vi "spectral_response_main.vi"() -> ()   [LabVIEW 2018]
uses:
  typedefs/measurement_settings.ctl
  typedefs/device_details.ctl
  typedefs/state_selector.ctl
  <instrlib>/Stanford Research 830/Stanford Research 830.lvlib
panel:
  in  "Monochromator Addr in":string="ASRL7::INSTR"
  out "white bias (# of suns)":dbl
  out "integrated jsc (mA/cm^2)":dbl
  out "Application Directory":path
  out "Application Directory":string
  out "Pixel scan number":string
  out "Scan number":string
  out "Pixel data file":path
  out "Ref data filepath":path
  in  "Tab Control":enum32{"Settings", "Measurement", "Advanced"}(tab)
  in  "Load measurement settings":bool
  in  "Save device details":bool
  in  "Load device details":bool
  in  "Measurement settings":T1={"Start Wavelength (nm)"=350.0, "End Wavelength (nm)"=900.0, "Increment (nm)"=5.0, "White Bias (No. of Suns)"=1.0, "Averages per wavlength"=5.0, "Time Constant"=8, "Low Pass Filter Slope "=1, "Gain (V/A)"=50.0} {"Gain (V/A)" format="%#.2f"; "Low Pass Filter Slope" items=["6 dB/oct", "12 dB/oct", "18 db/oct", "24 dB/oct"]; "Time Constant" items=["10 us", "30 us", "100 us", "300 us", "1 ms", "3 ms", "10 ms", "30 ms", "100 ms", "300 ms", "1 s", "3 s", "10 s", "30 s", "100 s", "300 s", "1 ks", "3 ks", "10 ks", "30 ks"]; "Averages per wavlength" format="%#.2f"; "White Bias (No. of Suns)" format="%#.2f"; "End Wavelength (nm)" min=350.0 max=1100.0 format="%#.2f"; "Start Wavelength (nm)" min=350.0 max=1100.0 format="%#.2f"}
  in  "Device details":T2={"Device label"="", "Experiment Variable"="", "Variable Value"="", "Pixel"=enum."1"}
  in  "Save measurement settings":bool
  out "Username":string
  out "Experiment Name":string
  out "Zero position set":bool
  in  "Scan":bool
  in  "Initialise instruments":bool
  in  "Find Zero":bool
  in  "Calibrate ref diode":bool
  in  "Stop scan":bool
  out "TTi Power Supply":bool
  out "Pixel Selector":bool
  out "Translation Stage":bool
  out "Monochromator":bool
  in  "Exit":bool
  out "Lock-in Amplifier":bool
  out "Reference measured":bool
  in  "Stop reference":bool
  in  "Wavelength (nm)":dbl
  in  "LED current (A)":dbl=0.1 min=0.0 max=0.5
  in  "Pixel":u16=1
  out "Light on":bool
  in  "Toggle white light":bool
  in  "Lock-in address":refnum<visa-resource-name>="GPIB0::8::INSTR"
  in  "TTi QL564P":refnum<visa-resource-name>="COM6"
  in  "Set wavelenth":bool
  in  "Set switch":bool
  in  "Input Connection (0: Single-Ended Voltage)":u16(ring) items=["Single-Ended Voltage", "Differential Voltage", "1 MOhm Current Gain", "100 MOhm Current Gain"]
  in  "Tab Control 2":enum32{"Page 1"}(tab)
  out "Graph":cluster{dbl[], "eqe measurements":dbl[]}[](graph)
  out "Graph 2":cluster{dbl[], dbl[]}(graph)
  # "Spectral Response Measurement"
  # "1."
  # "2."
  # "3."
  # "4."
  # "5."
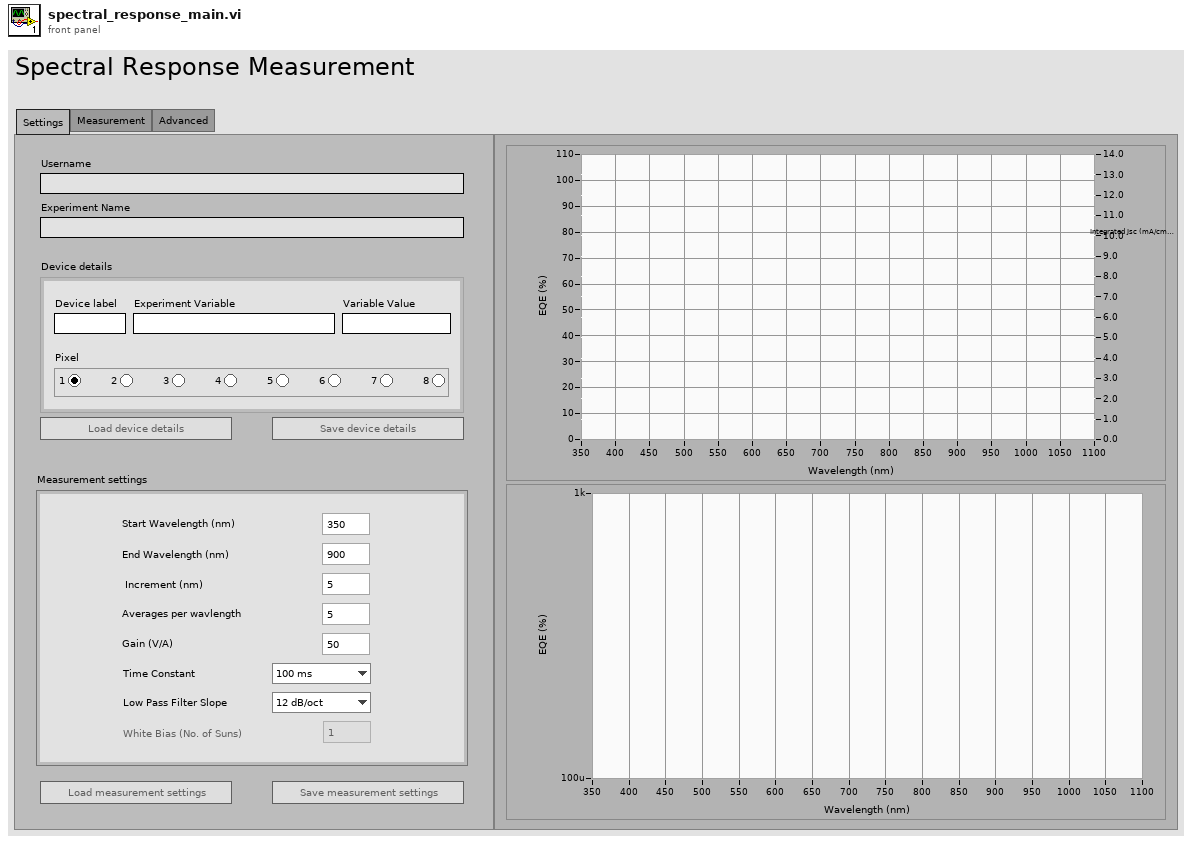
[diagram p1: front panel]
types:
  T1 = typedef "measurement_settings.ctl" = cluster{"Start Wavelength (nm)":dbl, "End Wavelength (nm)":dbl, "Increment (nm)":dbl, "White Bias (No. of Suns)":dbl, "Averages per wavlength":dbl, "Time Constant":u16, "Low Pass Filter Slope ":u16, "Gain (V/A)":dbl}
  T2 = typedef "device_details.ctl" = cluster{"Device label":string, "Experiment Variable":string, "Variable Value":string, "Pixel":enum32{"No Selection", "1", "2", "3", "4", "5", "6", "7", "8"}}
  T3 = typedef "state_selector.ctl" = enum16{"Initialise software", "Idle", "Load device details", "Save device details", "Initialise instruments", "Find zero position", "Calibrate ref diode", "Scan", "Exit"}
  T4 = enum8{"Enabled", "Disabled", "Disabled and Grayed Out"}
  T5 = cluster{"Device label":string, "Experiment Variable":string, "Variable Value":string, "Pixel":enum32{"No Selection", "1", "2", "3", "4", "5", "6", "7", "8"}}
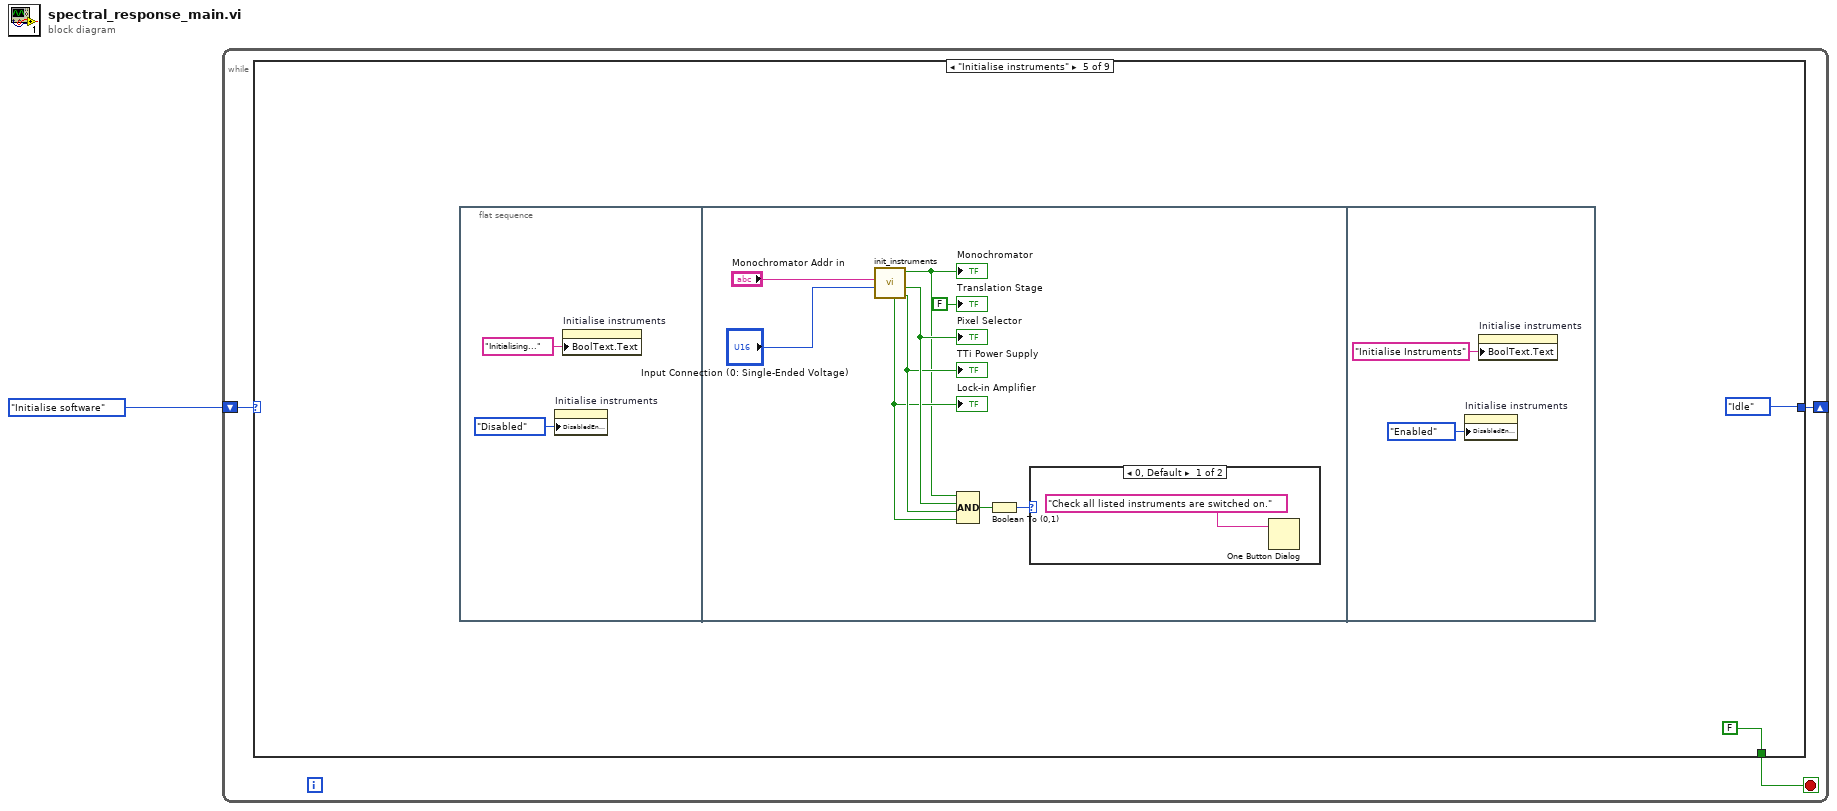
[diagram p0: block diagram]
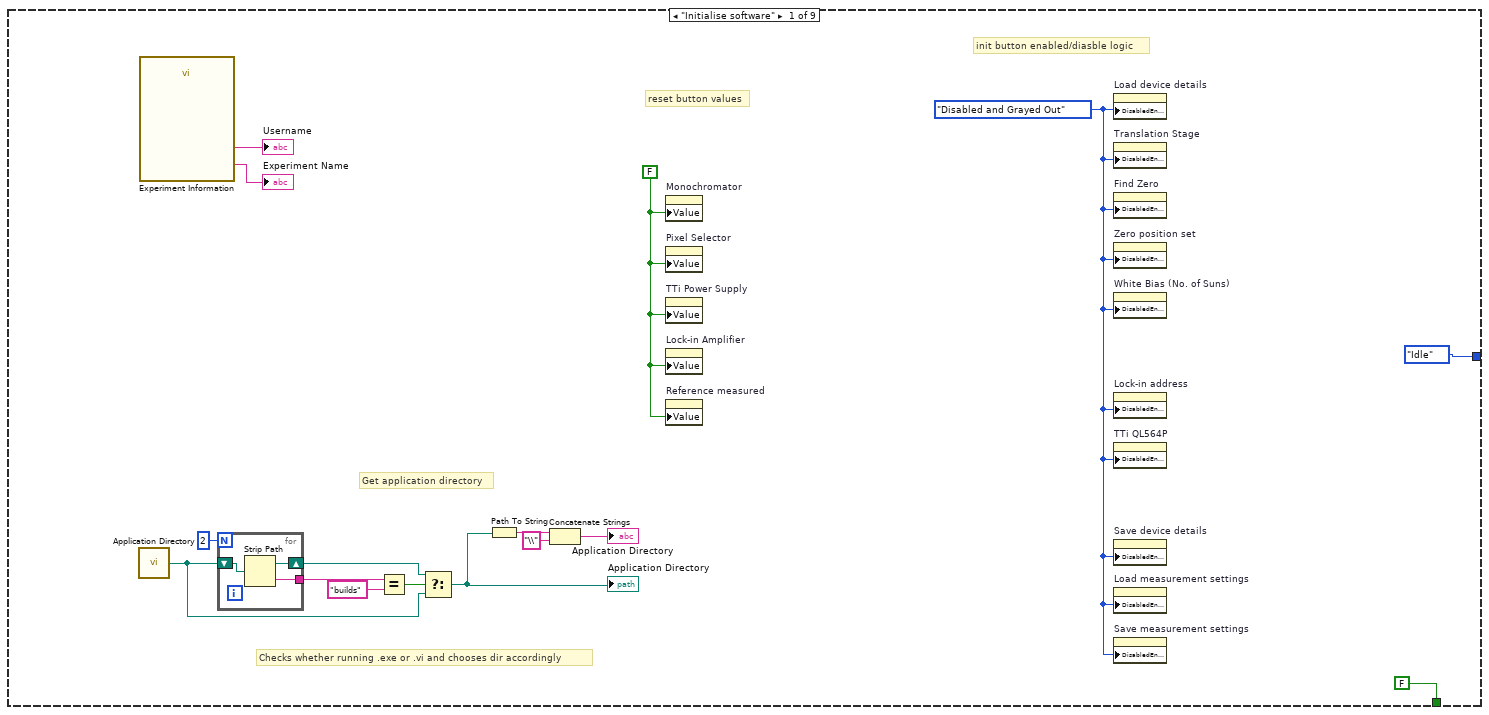
[diagram p2: hidden frame]
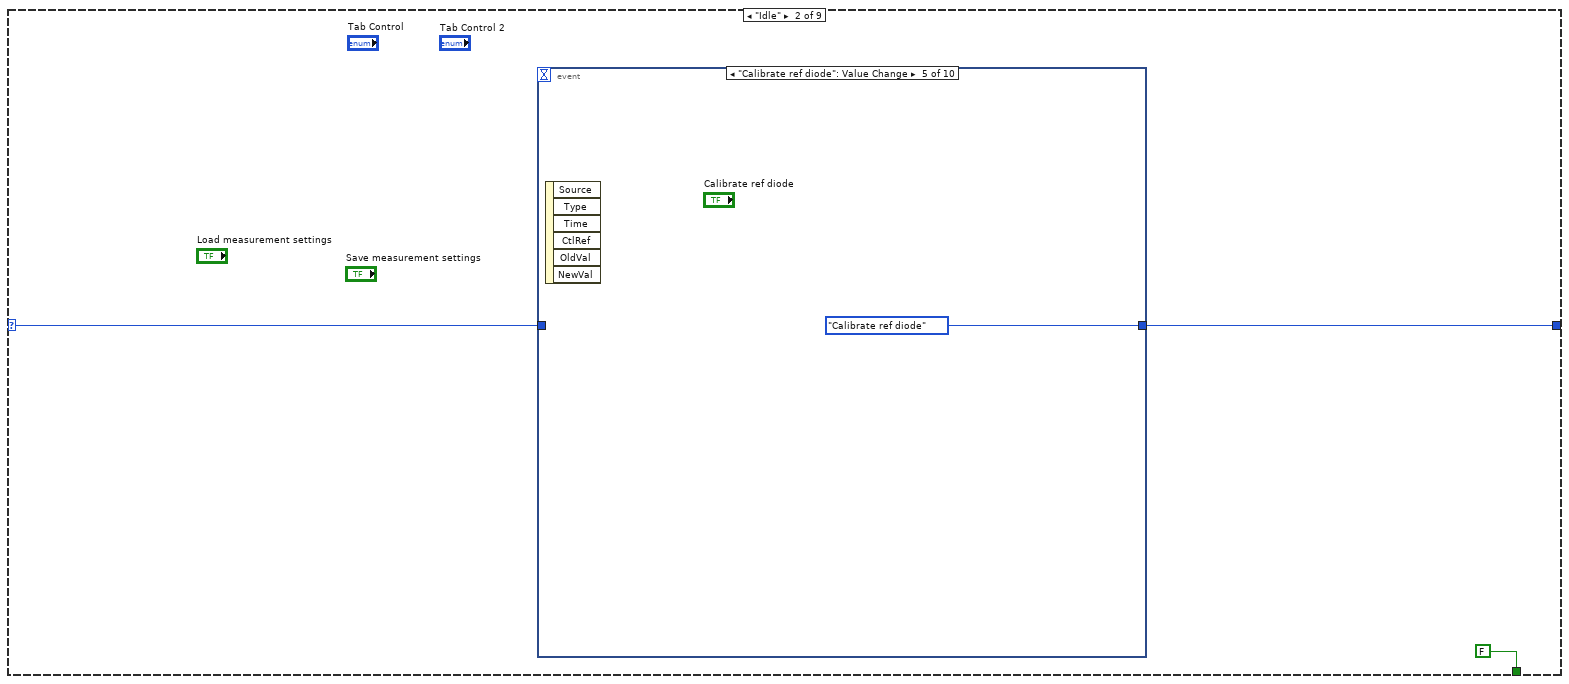
[diagram p3: hidden frame]
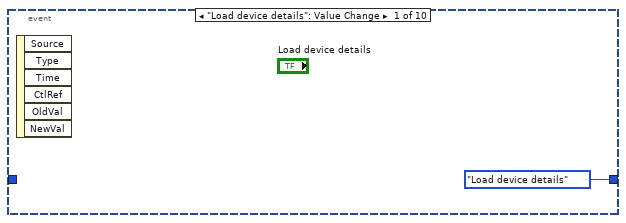
[diagram p4: hidden frame]
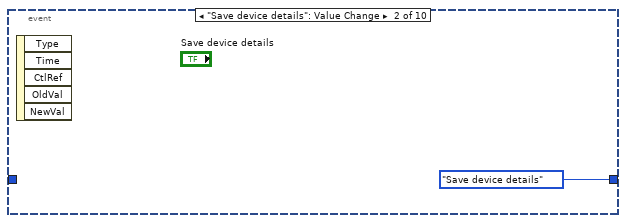
[diagram p5: hidden frame]
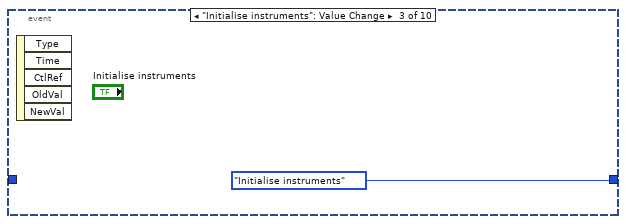
[diagram p6: hidden frame]
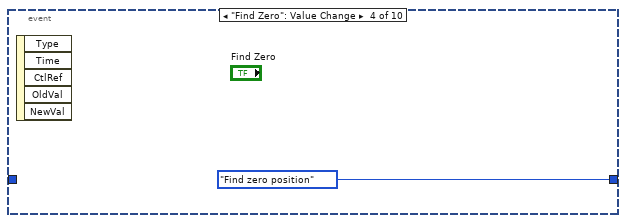
[diagram p7: hidden frame]
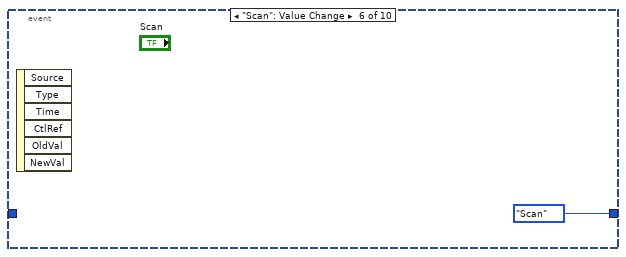
[diagram p8: hidden frame]
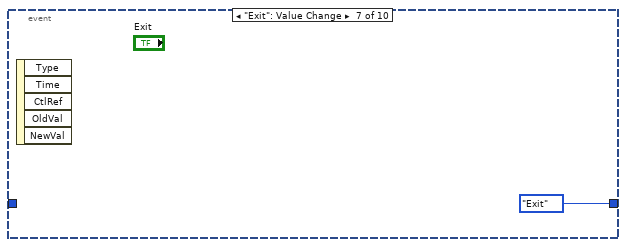
[diagram p9: hidden frame]
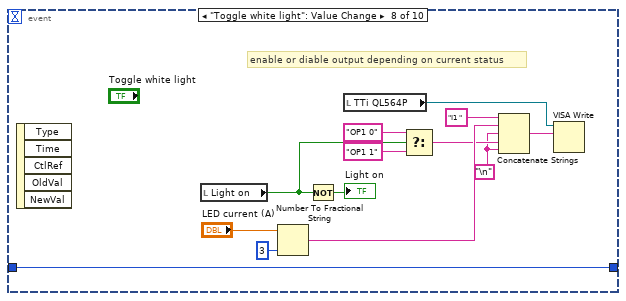
[diagram p10: hidden frame]
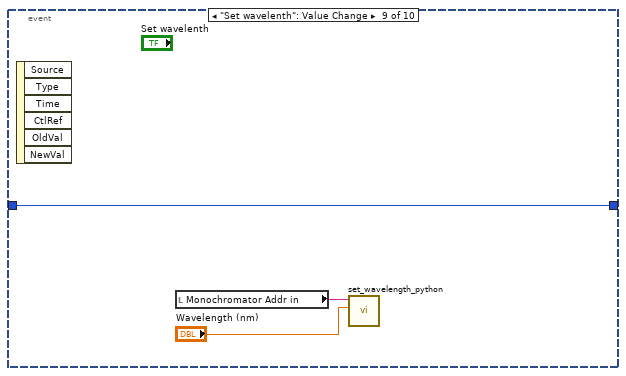
[diagram p11: hidden frame]
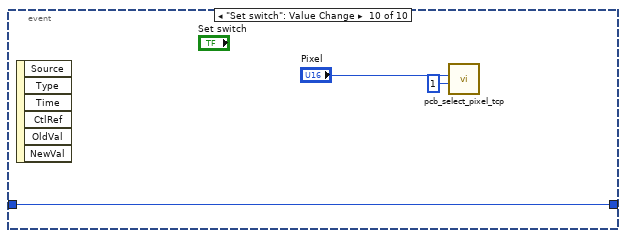
[diagram p12: hidden frame]
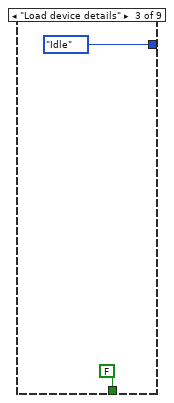
[diagram p13: hidden frame]
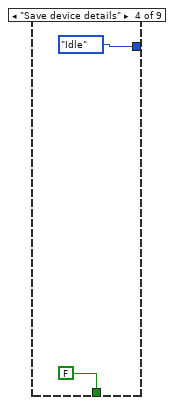
[diagram p14: hidden frame]
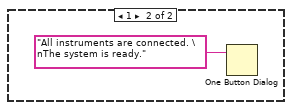
[diagram p15: hidden frame]
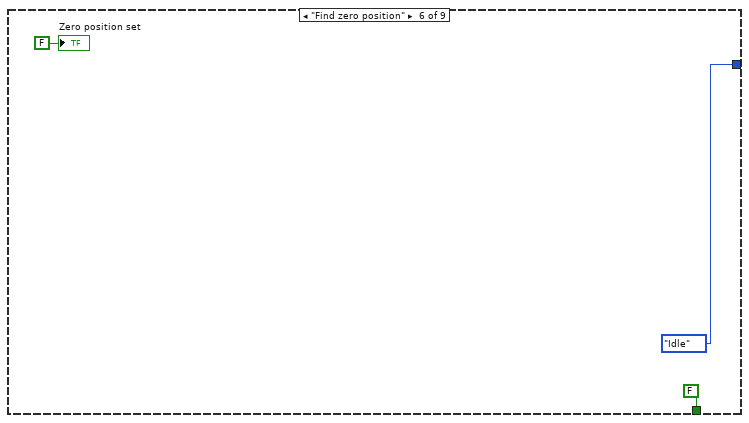
[diagram p16: hidden frame]
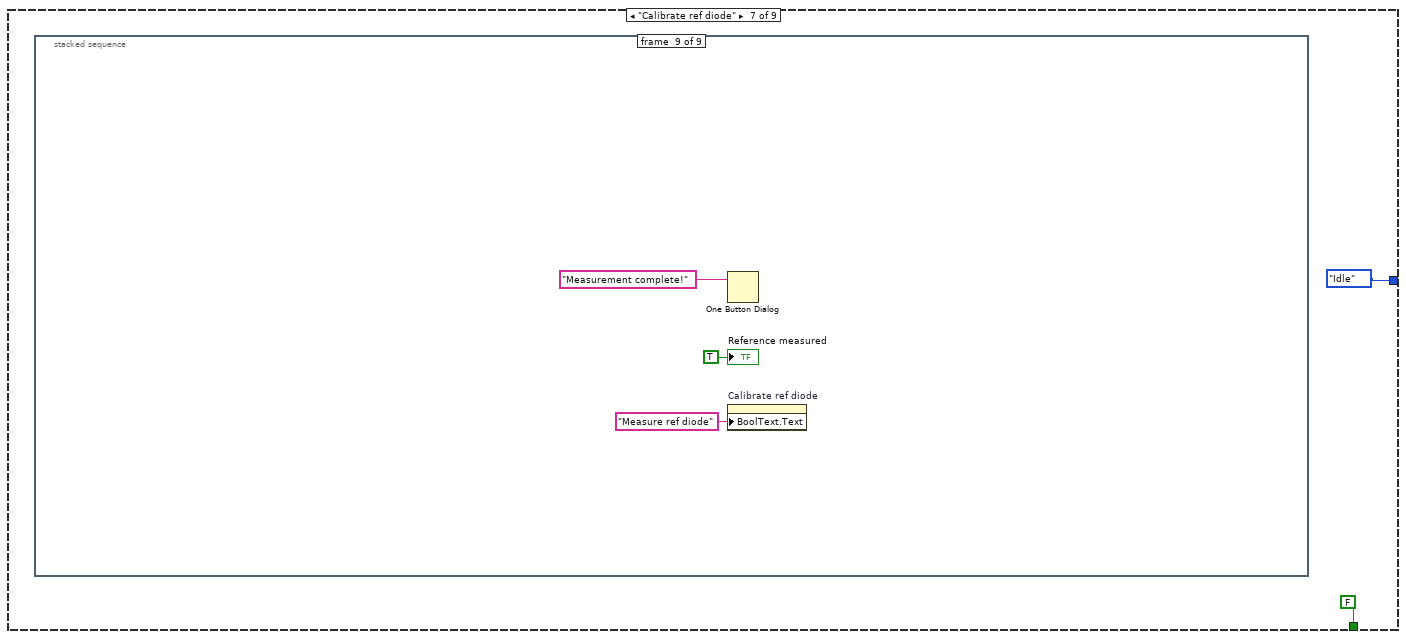
[diagram p17: hidden frame]
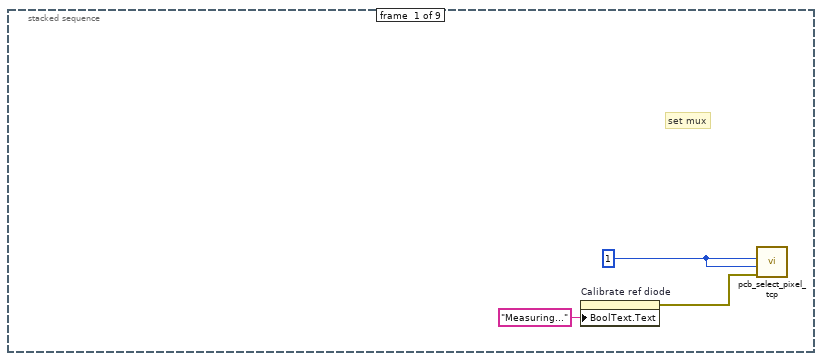
[diagram p18: hidden frame]
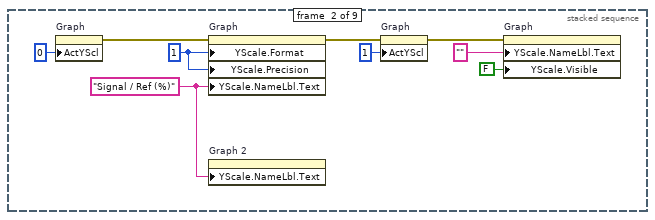
[diagram p19: hidden frame]
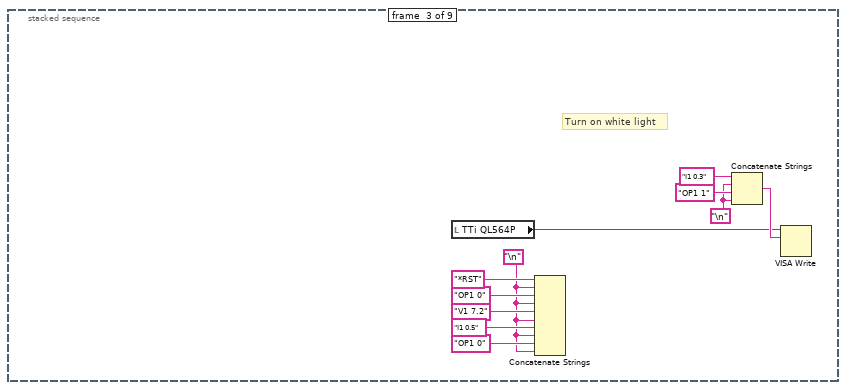
[diagram p20: hidden frame]
diagram:
  n1 = while {
    shift-right: [w3] -> _
    shift-left: state_selector."Initialise software" ("Enum") -> [w4]
    stop <- w2 stop-if-true
    n2 = case shown="\"Initialise instruments\"" w4 {
      selector: w4 -> [_ w25 _ _ _ _ _ _ _]
      tunnel: [state_selector."Idle" ("Enum") w26 state_selector."Idle" ("Enum") state_selector."Idle" ("Enum") state_selector."Idle" ("Enum") state_selector."Idle" ("Enum") state_selector."Idle" ("Enum") state_selector."Idle" ("Enum") state_selector."Exit" ("Enum")] -> w3
      tunnel: [FALSE FALSE FALSE FALSE FALSE FALSE FALSE FALSE TRUE] -> w2
      frame "Initialise software" {
        w15 = T4."Disabled and Grayed Out" ("Disabled")
        w16 = FALSE ("Scan")
        # "Checks whether running .exe or .vi and chooses dir accordingly"
        # "Get application directory"
        # "init button enabled/diasble logic"
        # "reset button values"
        n3 = call <vilib>:"Application Directory.vi"() -> ("Application Directory"=w6:path)
        n4 = call "Experiment Information"() -> ("Experiment Title"=→"Experiment Name":string, "Username"=→"Username":string)  [unwired: 16 in, 2 out]
        n5 = for {
          N: 2 -> [_]
          tunnel: [w21] -> w10
          shift-right: [w22] -> w7
          shift-left: w6 -> [w23]
          n6 = Strip Path(path=w23) -> (stripped path=w22:path, name=w21:string)
        }
        n7 = Equal?(x=w10, y="builds") -> (x = y?=w8:bool)
        n8 = Select(t=w7, s=w8, f=w6) -> (s? t:f=w5:path)
        "Application Directory" <- w5
        n9 = Path To String(path=w5) -> (string=w14:string)
        n10 = Concatenate Strings(w14, "\\" ("string")) -> (→"Application Directory":string)
        n11 = property on="Monochromator" class="Bool (strict)"("Value"=w16) -> ()  [unwired: 2 in, 2 out]
        n12 = property on="Pixel Selector" class="Bool (strict)"("Value"=w16) -> ()  [unwired: 2 in, 2 out]
        n13 = property on="TTi Power Supply" class="Bool (strict)"("Value"=w16) -> ()  [unwired: 2 in, 2 out]
        n14 = property on="Lock-in Amplifier" class="Bool (strict)"("Value"=w16) -> ()  [unwired: 2 in, 2 out]
        n15 = property on="Reference measured" class="Bool (strict)"("Value"=w16) -> ()  [unwired: 2 in, 2 out]
        n16 = property on="Load device details" class="Bool"("DisabledEnum"=w15) -> ()  [unwired: 2 in, 2 out]
        n17 = property on="Translation Stage" class="Bool (strict)"("DisabledEnum"=w15) -> ()  [unwired: 2 in, 2 out]
        n18 = property on="Find Zero" class="Bool"("DisabledEnum"=w15) -> ()  [unwired: 2 in, 2 out]
        n19 = property on="Zero position set" class="Bool (strict)"("DisabledEnum"=w15) -> ()  [unwired: 2 in, 2 out]
        n20 = property on="White Bias (No. of Suns)" class="DigNum (strict)"("DisabledEnum"=w15) -> ()  [unwired: 2 in, 2 out]
        n21 = property on="Lock-in address" class="VISAName"("DisabledEnum"=w15) -> ()  [unwired: 2 in, 2 out]
        n22 = property on="TTi QL564P" class="VISAName"("DisabledEnum"=w15) -> ()  [unwired: 2 in, 2 out]
        n23 = property on="Save device details" class="Bool"("DisabledEnum"=w15) -> ()  [unwired: 2 in, 2 out]
        n24 = property on="Load measurement settings" class="Bool"("DisabledEnum"=w15) -> ()  [unwired: 2 in, 2 out]
        n25 = property on="Save measurement settings" class="Bool"("DisabledEnum"=w15) -> ()  [unwired: 2 in, 2 out]
      }
      frame "Idle" {
        n26 = event shown="[4] \"Calibrate ref diode\": Value Change" {
          selector: _ -> [_ _ _ _ _ _ _ _ _ _]
          dyn-events: _ -> [_ _ _ _ _ _ _ _ _ _]
          timeout: _ -> [_ _ _ _ _ _ _ _ _ _]
          tunnel: w25 -> [_ _ _ _ _ _ _ w46 w49 w52]
          tunnel: [state_selector."Load device details" ("Enum") state_selector."Save device details" ("Enum") state_selector."Initialise instruments" ("Enum") state_selector."Find zero position" ("Enum") state_selector."Calibrate ref diode" ("Enum") state_selector."Scan" ("Enum") state_selector."Exit" ("Enum") w46 w49 w52] -> w26
          event "Load device details": Value Change {
            n27 = event-data() -> ()  [unwired: 1 in, 6 out]
          }
          event "Save device details": Value Change {
            n28 = event-data() -> ()  [unwired: 1 in, 5 out]
          }
          event "Initialise instruments": Value Change {
            n29 = event-data() -> ()  [unwired: 1 in, 5 out]
          }
          event "Find Zero": Value Change {
            n30 = event-data() -> ()  [unwired: 1 in, 5 out]
          }
          event "Calibrate ref diode": Value Change {
            n31 = event-data() -> ()  [unwired: 1 in, 6 out]
          }
          event "Scan": Value Change {
            n32 = event-data() -> ()  [unwired: 1 in, 6 out]
          }
          event "Exit": Value Change {
            n33 = event-data() -> ()  [unwired: 1 in, 5 out]
          }
          event "Toggle white light": Value Change {
            w34 = "\n"
            # "enable or diable output depending on current status"
            n34 = event-data() -> ()  [unwired: 1 in, 5 out]
            n35 = local read "Light on"() -> (w41:bool)
            n36 = Number To Fractional String(number="LED current (A)", precision (6)=i16 3) -> (F-format string=w37:string)  [unwired: 2 in]
            n37 = Not(x=w41) -> (.not. x?=→"Light on":bool)
            n38 = local read "TTi QL564P"() -> (w40:refnum<visa-resource-name>)
            n39 = Select(t="OP1 0" ("Channel Name"), s=w41, f="OP1 1" ("Channel Name")) -> (s? t:f=w35:string)
            n40 = Concatenate Strings("I1 " ("Channel Name"), w37, w34, w35, w34) -> (w45:string)
            n41 = VISA Write(VISA resource name=w40, write buffer=w45) -> ()  [unwired: 1 in, 3 out]
          }
          event "Set wavelenth": Value Change {
            n42 = event-data() -> ()  [unwired: 1 in, 6 out]
            n43 = local read "Monochromator Addr in"() -> (w48:string)
            n44 = call "set_wavelength_python.vi"("wavelength"="Wavelength (nm)", "Addr"=w48) -> ()  [unwired: 8 in, 2 out]
          }
          event "Set switch": Value Change {
            n45 = event-data() -> ()  [unwired: 1 in, 6 out]
            n46 = call "pcb_select_pixel_tcp.vi"("Cell"=u32 1, "Pixel"="Pixel") -> ()  [unwired: 8 in, 2 out]
          }
        }
      }
      frame "Load device details" {
      }
      frame "Save device details" {
      }
      frame "Initialise instruments" {
        n47 = flat-sequence {
          frame #0 {
            n48 = property on="Initialise instruments" class="Bool"("DisabledEnum"=T4."Disabled" ("Disabled")) -> ()  [unwired: 2 in, 2 out]
            n49 = property on="Initialise instruments" class="Bool"("BoolText.Text"="Initialising..." ("Boolean Text.Text")) -> ()  [unwired: 2 in, 2 out]
          }
          frame #1 {
            n50 = call "init_instruments.vi"("Input Connection (0: Single-Ended Voltage)"="Input Connection (0: Single-Ended Voltage)", "Monochromator Addr in"="Monochromator Addr in") -> ("LED power supply"=w66:bool, "Pixel Selector"=w67:bool, "Monochromator"=w64:bool, "Lock-in amplifier"=w65:bool)  [unwired: 6 in]
            "Lock-in Amplifier" <- w65
            "Monochromator" <- w64
            "Pixel Selector" <- w67
            "TTi Power Supply" <- w66
            n51 = Compound Arithmetic op=AND(w64, w67, w66, w65) -> (w69:bool)
            n52 = Boolean To (0,1)(Boolean=w69) -> (0, 1=w68:i16)
            n53 = case shown="0, Default" w68 {
              frame 0, Default {
                n54 = One Button Dialog(message="Check all listed instruments are switched on.") -> ()  [unwired: 1 in, 1 out]
              }
              frame 1 {
                n55 = One Button Dialog(message="All instruments are connected. \nThe system is ready.") -> ()  [unwired: 1 in, 1 out]
              }
            }
            "Translation Stage" <- FALSE ("Translation Stage")
          }
          frame #2 {
            n56 = property on="Initialise instruments" class="Bool"("DisabledEnum"=T4."Enabled" ("Disabled")) -> ()  [unwired: 2 in, 2 out]
            n57 = property on="Initialise instruments" class="Bool"("BoolText.Text"="Initialise Instruments" ("Boolean Text.Text")) -> ()  [unwired: 2 in, 2 out]
          }
        }
      }
      frame "Find zero position" {
        "Zero position set" <- FALSE ("Zero position set")
      }
      frame "Calibrate ref diode" {
        n58 = stacked-sequence {
          frame #0 {
            w79 = u32 1 ("Pixel")
            # "set mux"
            n59 = property on="Calibrate ref diode" class="Bool"("BoolText.Text"="Measuring..." ("Boolean Text.Text")) -> (error out=w80:errorcluster)  [unwired: 2 in, 1 out]
            n60 = call "pcb_select_pixel_tcp.vi"("error in (no error)"=w80, "Cell"=w79, "Pixel"=w79) -> ()  [unwired: 7 in, 2 out]
          }
          frame #1 {
            w86 = u8 1 ("Y Scale.Display Format:Format")
            w85 = "Signal / Ref (%)" ("Y Scale.Name Label.Text")
            n61 = property on="Graph" class="XYGraph (strict)"("ActYScl"=0 ("Active Y Scale")) -> (error out=w84:errorcluster)  [unwired: 2 in, 1 out]
            n62 = property on="Graph" class="XYGraph (strict)"(error in=w84, "YScale.Format"=w86, "YScale.Precision"=w86, "YScale.NameLbl.Text"=w85) -> (error out=w83:errorcluster)  [unwired: 1 in, 1 out]
            n63 = property on="Graph 2" class="XYGraph (strict)"("YScale.NameLbl.Text"=w85) -> ()  [unwired: 2 in, 2 out]
            n64 = property on="Graph" class="XYGraph (strict)"(error in=w83, "ActYScl"=1 ("Active Y Scale")) -> (error out=w87:errorcluster)  [unwired: 1 in, 1 out]
            n65 = property on="Graph" class="XYGraph (strict)"(error in=w87, "YScale.NameLbl.Text"="" ("Y Scale.Name Label.Text"), "YScale.Visible"=FALSE ("Y Scale.Visible")) -> ()  [unwired: 1 in, 2 out]
          }
          frame #2 {
            w92 = "\n"
            w96 = "\n"
            # "Turn on white light"
            n66 = local read "TTi QL564P"() -> (w91:refnum<visa-resource-name>)
            n67 = Concatenate Strings("*RST" ("string"), w96, "OP1 0" ("string"), w96, "V1 7.2" ("string"), w96, "I1 0.5" ("string"), w96, "OP1 0" ("string"), w96) -> ()  [unwired: 1 out]
            n68 = Concatenate Strings("I1 0.3" ("string"), w92, "OP1 1" ("string"), w92) -> (w95:string)
            n69 = VISA Write(VISA resource name=w91, write buffer=w95) -> ()  [unwired: 1 in, 3 out]
          }
          frame #3 {
            # "save data"
            # "Create list of wavelengths"
            n70 = local read "Measurement settings"() -> (w117:T1)
            n71 = local read "Lock-in address"() -> (w105:refnum<visa-resource-name>)
            n72 = Unbundle By Name(w117) -> ("Time Constant"=w107:u16, "Low Pass Filter Slope"=w106:u16)
            n73 = local read "Monochromator Addr in"() -> (w102:string)
            n74 = call "create_wavelength_array.vi"("Measurement settings"=w117) -> ("wavelengths array"=w125:dbl[])  [unwired: 9 in, 1 out]
            n75 = call <instrlib>:"Configure Filter.vi"("Enable Sync Filter (F: Disable)"=FALSE ("Enable Sync Filter"), "error in (no error)"=errorcluster {"status"=FALSE, "code"=0, "source"=""} ("error out"), "Low Pass Filter Slope (1: 12dB/oct)"=w106, "Time Constant (8: 100ms)"=w107, "VISA resource name"=w105) -> ("error out"=w103:errorcluster, "VISA resource name out"=w108:refnum<visa-resource-name>)  [unwired: 5 in]
            n76 = for {
              tunnel: w125 -> [w126] mode=indexing
              shift-right: [w142] -> _
              shift-left: w103 -> [w129]
              tunnel: w117 -> [w141]
              shift-right: [w136] -> w121
              shift-left: dbl[] [] -> [w139]
              shift-right: [w137] -> w122
              shift-left: dbl[] [] -> [w138]
              tunnel: w108 -> [w133]
              tunnel: w102 -> [w127]
              stop <- "Stop reference" stop-if-true
              # "Meas I"
              # "Set wl"
              n77 = call "set_wavelength_python.vi"("error in (no error)"=w129, "wavelength"=w126, "Addr"=w127) -> ("error out"=w128:errorcluster)  [unwired: 7 in, 1 out]
              n78 = call "determine_gain.vi"("error in (no error)"=w128, "VISA resource name"=w133) -> ("error out"=w132:errorcluster, "VISA resource name out"=w134:refnum<visa-resource-name>)  [unwired: 8 in]
              n79 = call "measure_ratio_signal.vi"("error in"=w132, "Measurement settings"=w141, "VISA resource name in"=w134) -> ("error out"=w142:errorcluster, "Averaged scaled ratio"=w140:dbl)  [unwired: 6 in, 1 out]
              n80 = Insert Into Array(array=w139, new element=w140) -> (w136:dbl[])  [unwired: 1 in]
              n81 = Insert Into Array(array=w138, new element=w126) -> (w137:dbl[])  [unwired: 1 in]
              n82 = Bundle(w137, w136) -> (w130:cluster{dbl[], dbl[]})  [unwired: 1 in]
              n83 = Build Array(w130) -> (w131:cluster{dbl[], dbl[]}[])
              n84 = local write "Graph 2"(w130) -> ()
              n85 = local write "Graph"(w131) -> ()
            }
            n86 = local read "Application Directory"() -> (w110:string)
            n87 = local read "Username"() -> (w112:string)
            n88 = local read "Experiment Name"() -> (w113:string)
            n89 = Build Array(w122, w121) -> (w120:dbl[][])
            n90 = Transpose 2D Array(2D array=w120) -> (transposed array=w118:dbl[][])
            n91 = call "create_data_file.vi"("Application Directory"=w110, "Pixel"="", "Device label"="ref_diode", "Experiment Title"=w113, "Username"=w112) -> ("Scan number"=→"Scan number":string, "Filepath out"=w116:path)  [unwired: 5 in]
            n92 = call "save_data.vi"("wl-current array"=w118, "Application Directory"=w110, "Filepath in"=w116) -> ("Filepath out"=→"Ref data filepath":path)  [unwired: 8 in]
          }
          frame #4 {
            # "Turn off white light"
            n93 = local read "TTi QL564P"() -> (w143:refnum<visa-resource-name>)
            n94 = Concatenate Strings("OP1 0" ("Channel Name"), "\n") -> (w145:string)
            n95 = VISA Write(VISA resource name=w143, write buffer=w145) -> ()  [unwired: 1 in, 3 out]
          }
          frame #5 {
            # "Add measurement info to log file"
            n96 = local read "Application Directory"() -> (w157:string)
            n97 = local read "Lock-in address"() -> (w147:refnum<visa-resource-name>)
            n98 = local read "Ref data filepath"() -> (w163:path)
            n99 = local read "Username"() -> (w161:string)
            n100 = local read "Experiment Name"() -> (w160:string)
            n101 = local read "Measurement settings"() -> (w162:T1)
            n102 = local read "Scan number"() -> (w158:string)
            n103 = call "SR830_any.vi"("initial string"="OFLT? ", "VISA resource name"=w147) -> ("Measurement"=w150:dbl)  [unwired: 7 in, 2 out]
            n104 = call "sr830_convert_time_constant.vi"("Time constant code"=w150) -> ("time constant  in ms"=w149:dbl)  [unwired: 2 in]
            n105 = call "SR830_any.vi"("initial string"="FREQ? ", "VISA resource name"=w147) -> ("Measurement"=w153:dbl)  [unwired: 7 in, 2 out]
            n106 = Number To Fractional String(number=w149) -> (F-format string=w148:string)  [unwired: 3 in]
            n107 = Number To Fractional String(number=w153) -> (F-format string=w152:string)  [unwired: 3 in]
            n108 = call "create_save_log_file.vi"("Username"=w161, "Data filepath"=w163, "Frequency (Hz)"=w152, "Application Directory"=w157, "Experiment Title"=w160, "Time constant (ms)"=w148, "Device details"=T5 {"Device label"="ref_diode", "Experiment Variable"="n/a", "Variable Value"="n/a", "Pixel"=enum."1"} ("Device details 2"), "Measurement settings"=w162, "Scan number"=w158, "white bias (# of suns)"=1.0 ("integrated jsc (mA/cm^2)"), "integrated jsc (mA/cm^2)"=0.0) -> ()  [unwired: 4 in, 1 out]
          }
          frame #6 {
            w165 = i16 26 items=["Auto Gain"=-1, "2 nV/fA"=0, "5 nV/fA"=1, "10 nV/fA"=2, "20 nV/fA"=3, "50 nV/fA"=4, "100 nV/fA"=5, "200 nV/fA"=6, "500 nV/fA"=7, "1 uV/pA"=8, "2 uV/pA"=9, "5 uV/pA"=10, "10 uV/pA"=11, "20 uV/pA"=12, "50 uV/pA"=13, "100 uV/pA"=14, "200 uV/pA"=15, "500 uV/pA"=16, "1 mV/nA"=17, "2 mV/nA"=18, "5 mV/nA"=19, "10 mV/nA"=20, "20 mV/nA"=21, "50 mV/nA"=22, "100 mV/nA"=23, "200 mV/nA"=24, "500 mV/mA"=25, "1 V/uA"=26] ("Sensitivity (-1: Auto gain)")
            w166 = i16 -1 items=["Auto Reserve"=-1, "High Reserve"=0, "Normal"=1, "Low Noise"=2] ("Dynamic Reserve (-1: Auto Reserve)")
            n109 = local read "Lock-in address"() -> (w164:refnum<visa-resource-name>)
            n110 = call <instrlib>:"Configure Sensitivity and Reserve.vi"("Sensitivity (-1: Auto gain)"=w165, "Dynamic Reserve (-1: Auto Reserve)"=w166, "VISA resource name"=w164) -> ()  [unwired: 7 in, 2 out]
          }
          frame #7 {
            # "Reset wavelength to 550nm"
            n111 = local read "Monochromator Addr in"() -> (w168:string)
            n112 = call "set_wavelength_python.vi"("wavelength"=550.0, "Addr"=w168) -> ()  [unwired: 8 in, 2 out]
          }
          frame #8 {
            n113 = One Button Dialog(message="Measurement complete!") -> ()  [unwired: 1 in, 1 out]
            n114 = property on="Calibrate ref diode" class="Bool"("BoolText.Text"="Measure ref diode" ("Boolean Text.Text")) -> ()  [unwired: 2 in, 2 out]
            "Reference measured" <- TRUE ("Calibration completed")
          }
        }
      }
      frame "Scan" {
        n115 = stacked-sequence {
          frame #0 {
            # "Set mux"
            n116 = property on="Scan" class="Bool"("BoolText.Text"="Measuring..." ("Boolean Text.Text")) -> (error out=w176:errorcluster)  [unwired: 2 in, 1 out]
            n117 = call "get_pixel_number.vi"("Device details"="Device details") -> ("Pixel"=w175:i32)  [unwired: 9 in, 1 out]
            n118 = call "pcb_select_pixel_tcp.vi"("error in (no error)"=w176, "Cell"=u32 1, "Pixel"=w175) -> ()  [unwired: 7 in, 2 out]
          }
          frame #1 {
            w182 = u8 0 ("Y Scale.Display Format:Format")
            w183 = "EQE (%)" ("Y Scale.Name Label.Text")
            n119 = property on="Graph" class="XYGraph (strict)"("ActYScl"=0 ("Active Y Scale")) -> (error out=w189:errorcluster)  [unwired: 2 in, 1 out]
            n120 = property on="Graph" class="XYGraph (strict)"(error in=w189, "YScale.Format"=w182, "YScale.Precision"=w182, "YScale.NameLbl.Text"=w183) -> (error out=w187:errorcluster)  [unwired: 1 in, 1 out]
            n121 = property on="Graph 2" class="XYGraph (strict)"("YScale.NameLbl.Text"=w183) -> ()  [unwired: 2 in, 2 out]
            n122 = property on="Graph" class="XYGraph (strict)"(error in=w187, "ActYScl"=1 ("Active Y Scale")) -> (error out=w184:errorcluster)  [unwired: 1 in, 1 out]
            n123 = property on="Graph" class="XYGraph (strict)"(error in=w184, "YScale.Format"=u8 0 ("Y Scale.Display Format:Format"), "YScale.Precision"=u8 1 ("Y Scale.Display Format:Precision"), "YScale.NameLbl.Text"="Integrated Jsc (mA/cm^2)" ("Y Scale.Name Label.Text"), "YScale.Visible"=TRUE ("Y Scale.Visible")) -> ()  [unwired: 1 in, 2 out]
          }
          frame #2 {
            w192 = "\n"
            w198 = "\n"
            # "Turn on white ligth bias"
            n124 = Concatenate Strings("*RST" ("string"), w198, "OP1 0" ("string"), w198, "V1 7.2" ("string"), w198, "I1 0.5" ("string"), w198, "OP1 0" ("string"), w198) -> (w197:string)
            n125 = VISA Write(VISA resource name="TTi QL564P", write buffer=w197) -> (VISA resource name out=w191:refnum<visa-resource-name>, error out=w190:errorcluster)  [unwired: 1 in, 1 out]
            n126 = Concatenate Strings("I1 0.3" ("string"), w192, "OP1 1" ("string"), w192) -> (w195:string)
            n127 = VISA Write(VISA resource name=w191, write buffer=w195, error in (no error)=w190) -> ()  [unwired: 3 out]
          }
          frame #3 {
            w218 = FALSE  # Enable Sync Filter
            # "Save data"
            # "Scan pixel and save data"
            # "Create list of wavelengths"
            n128 = local read "Monochromator Addr in"() -> (w205:string)
            n129 = Unbundle By Name("Measurement settings") -> ("Time Constant"=w216:u16, "Low Pass Filter Slope"=w215:u16)
            n130 = call "create_wavelength_array.vi"("Measurement settings"="Measurement settings") -> ("wavelengths array"=w236:dbl[])  [unwired: 9 in, 1 out]
            n131 = call <instrlib>:"Configure Filter.vi"("Enable Sync Filter (F: Disable)"=w218, "error in (no error)"=errorcluster {"status"=FALSE, "code"=0, "source"=""} ("error out"), "Low Pass Filter Slope (1: 12dB/oct)"=w215, "Time Constant (8: 100ms)"=w216, "VISA resource name"="Lock-in address") -> ("error out"=w206:errorcluster, "VISA resource name out"=w217:refnum<visa-resource-name>)  [unwired: 5 in]
            n132 = local read "Application Directory"() -> (w204:string)
            n133 = for {
              tunnel: w236 -> [w238] mode=indexing
              shift-right: [w260] -> _
              shift-left: w206 -> [w241]
              tunnel: "Measurement settings" -> [w259]
              shift-right: [w254] -> w231
              shift-left: dbl[] [] -> [w257]
              shift-right: [w242] -> w232
              shift-left: dbl[] [] -> [w256]
              shift-right: [w243] -> w230
              shift-left: dbl[] [] -> [_]
              tunnel: w217 -> [w251]
              tunnel: w204 -> [w253]
              shift-right: [w245] -> w212
              shift-left: dbl[] [] -> [w249]
              tunnel: [w243] -> w211
              tunnel: [w242] -> w210
              tunnel: w205 -> [w239]
              tunnel: w204 -> [w237]
              stop <- "Stop scan" stop-if-true
              # "calculate cumulative Jsc"
              # "Calculate EQE from ref data"
              # "Meas I"
              # "Set wl"
              n134 = call "set_wavelength_python.vi"("error in (no error)"=w241, "wavelength"=w238, "Addr"=w239) -> ("error out"=w240:errorcluster)  [unwired: 7 in, 1 out]
              n135 = call "determine_gain.vi"("error in (no error)"=w240, "VISA resource name"=w251) -> ("error out"=w252:errorcluster, "VISA resource name out"=w250:refnum<visa-resource-name>)  [unwired: 8 in]
              n136 = call "measure_ratio_signal.vi"("error in"=w252, "Measurement settings"=w259, "VISA resource name in"=w250) -> ("error out"=w260:errorcluster, "Averaged scaled ratio"=w258:dbl)  [unwired: 6 in, 1 out]
              n137 = Insert Into Array(array=w257, new element=w258) -> (w254:dbl[])  [unwired: 1 in]
              n138 = Insert Into Array(array=w256, new element=w238) -> (w242:dbl[])  [unwired: 1 in]
              n139 = local read "Ref data filepath"() -> (w255:path)
              n140 = call "calculate_eqe.vi"("Application Directory"=w253, "wavelengths"=w242, "current measurements"=w254, "Ref data filepath"=w255) -> ("eqe measurements"=w243:dbl[])  [unwired: 7 in]
              n141 = call "calculate_jsc.vi"("Application Directory"=w237, "wavelengths"=w242, "eqe measurements"=w243) -> ("jsc (mA/cm^2)"=w248:dbl)  [unwired: 8 in]
              n142 = Insert Into Array(array=w249, new element=w248) -> (w245:dbl[])  [unwired: 1 in]
              n143 = Bundle(w242, "eqe measurements"=w243) -> (w247:cluster{dbl[], "eqe measurements":dbl[]})  [unwired: 1 in]
              "Graph 2" <- w247
              n144 = Bundle(w242, w245) -> (w244:cluster{dbl[], dbl[]})  [unwired: 1 in]
              n145 = Build Array(w247, w244) -> (→"Graph":cluster{dbl[], "eqe measurements":dbl[]}[])
            }
            n146 = local read "Username"() -> (w224:string)
            n147 = local read "Experiment Name"() -> (w223:string)
            n148 = local read "Device details"() -> (w227:T2)
            n149 = Build Array(w232, w231, w230, w212) -> (w229:dbl[][])
            n150 = Array Max & Min(array=w212) -> (max value=w209:dbl)  [unwired: 3 out]
            "integrated jsc (mA/cm^2)" <- w209
            n151 = Transpose 2D Array(2D array=w229) -> (transposed array=w228:dbl[][])
            n152 = call "calculate_white-bias_jsc.vi"("Application Directory"=w204, "wavelengths"=w210, "eqe measurements"=w211, "am1.5 jsc (mA/cm^2)"=w209) -> ("white bias (# of suns)"=→"white bias (# of suns)":dbl)  [unwired: 7 in]
            n153 = Unbundle By Name(w227) -> ("Device label"=w222:string)
            n154 = call "get_pixel_number.vi"("Device details"=w227) -> ("Pixel string"=w221:string)  [unwired: 9 in, 1 out]
            n155 = call "create_data_file.vi"("Application Directory"=w204, "Pixel"=w221, "Device label"=w222, "Experiment Title"=w223, "Username"=w224) -> ("Scan number"=→"Pixel scan number":string, "Filepath out"=w225:path)  [unwired: 5 in]
            n156 = call "save_data.vi"("wl-current array"=w228, "Application Directory"=w204, "Filepath in"=w225) -> ("Filepath out"=→"Pixel data file":path)  [unwired: 8 in]
          }
          frame #4 {
            # "Turn off white light"
            n157 = local read "TTi QL564P"() -> (w262:refnum<visa-resource-name>)
            n158 = Concatenate Strings("OP1 0" ("Channel Name"), "\n") -> (w264:string)
            n159 = VISA Write(VISA resource name=w262, write buffer=w264) -> ()  [unwired: 1 in, 3 out]
          }
          frame #5 {
            # "Save data to log file"
            n160 = local read "Application Directory"() -> (w276:string)
            n161 = local read "Lock-in address"() -> (w266:refnum<visa-resource-name>)
            n162 = local read "Pixel data file"() -> (w281:path)
            n163 = local read "Username"() -> (w282:string)
            n164 = local read "Experiment Name"() -> (w280:string)
            n165 = local read "Device details"() -> (w279:T2)
            n166 = local read "Measurement settings"() -> (w278:T1)
            n167 = local read "Pixel scan number"() -> (w277:string)
            n168 = local read "white bias (# of suns)"() -> (w274:dbl)
            n169 = local read "integrated jsc (mA/cm^2)"() -> (w275:dbl)
            n170 = call "SR830_any.vi"("initial string"="OFLT? ", "VISA resource name"=w266) -> ("Measurement"=w269:dbl)  [unwired: 7 in, 2 out]
            n171 = call "sr830_convert_time_constant.vi"("Time constant code"=w269) -> ("time constant  in ms"=w268:dbl)  [unwired: 2 in]
            n172 = Number To Fractional String(number=w268) -> (F-format string=w267:string)  [unwired: 3 in]
            n173 = call "SR830_any.vi"("initial string"="FREQ? ", "VISA resource name"=w266) -> ("Measurement"=w272:dbl)  [unwired: 7 in, 2 out]
            n174 = Number To Fractional String(number=w272) -> (F-format string=w271:string)  [unwired: 3 in]
            n175 = call "create_save_log_file.vi"("Username"=w282, "Data filepath"=w281, "Frequency (Hz)"=w271, "Application Directory"=w276, "Experiment Title"=w280, "Time constant (ms)"=w267, "Device details"=w279, "Measurement settings"=w278, "Scan number"=w277, "white bias (# of suns)"=w274, "integrated jsc (mA/cm^2)"=w275) -> ()  [unwired: 4 in, 1 out]
          }
          frame #6 {
            w285 = i16 20 items=["Auto Gain"=-1, "2 nV/fA"=0, "5 nV/fA"=1, "10 nV/fA"=2, "20 nV/fA"=3, "50 nV/fA"=4, "100 nV/fA"=5, "200 nV/fA"=6, "500 nV/fA"=7, "1 uV/pA"=8, "2 uV/pA"=9, "5 uV/pA"=10, "10 uV/pA"=11, "20 uV/pA"=12, "50 uV/pA"=13, "100 uV/pA"=14, "200 uV/pA"=15, "500 uV/pA"=16, "1 mV/nA"=17, "2 mV/nA"=18, "5 mV/nA"=19, "10 mV/nA"=20, "20 mV/nA"=21, "50 mV/nA"=22, "100 mV/nA"=23, "200 mV/nA"=24, "500 mV/mA"=25, "1 V/uA"=26] ("Sensitivity (-1: Auto gain)")
            w284 = i16 -1 items=["Auto Reserve"=-1, "High Reserve"=0, "Normal"=1, "Low Noise"=2] ("Dynamic Reserve (-1: Auto Reserve)")
            # "Set lock-in to not very sensitive range to prevent overload"
            n176 = local read "Lock-in address"() -> (w283:refnum<visa-resource-name>)
            n177 = call <instrlib>:"Configure Sensitivity and Reserve.vi"("Sensitivity (-1: Auto gain)"=w285, "Dynamic Reserve (-1: Auto Reserve)"=w284, "VISA resource name"=w283) -> ()  [unwired: 7 in, 2 out]
          }
          frame #7 {
            # "Reset wavelength to 550nm"
            n178 = local read "Monochromator Addr in"() -> (w287:string)
            n179 = call "set_wavelength_python.vi"("wavelength"=550.0, "Addr"=w287) -> ()  [unwired: 8 in, 2 out]
          }
          frame #8 {
            n180 = One Button Dialog(message="Measurement complete!") -> ()  [unwired: 1 in, 1 out]
            n181 = property on="Scan" class="Bool"("BoolText.Text"="Measure pixel" ("Boolean Text.Text")) -> ()  [unwired: 2 in, 2 out]
          }
        }
      }
      frame "Exit" {
        n182 = local read "TTi QL564P"() -> (w290:refnum<visa-resource-name>)
        n183 = VISA Clear(VISA resource name=w290) -> (VISA resource name out=w292:refnum<visa-resource-name>, error out=w291:errorcluster)  [unwired: 1 in]
        n184 = VISA Close(VISA resource name=w292, error in (no error)=w291) -> ()  [unwired: 1 out]
      }
    }
  }
